vi "Measurement Logic.vi"() -> ()   [LabVIEW 2021, in "audio_intermodulationDistortionMeasurement.lvlib"]
uses:
  audio_intermodulationDistortionMeasurement.lvlib
  <vilib>/MeasurementLink/MeasurementLink Measurement Server/Classes/MeasurementContext/MeasurementContext.lvclass
  <vilib>/PDM Acquisition Toolkit/host/Classes/Tasks/PCM Input/Controls/DVR PCM Input Task.ctl
  <vilib>/PDM Acquisition Toolkit/host/Classes/Tasks/PCM Input/PCM Input Task.lvclass
  <vilib>/DAQmx/create/channels.llb/DAQmx Create Channel (AO-Voltage-Basic).vi
  <vilib>/DAQmx/configure/timing.llb/DAQmx Timing (Sample Clock).vi
  <vilib>/PDM Acquisition Toolkit/host/API/Public/Start/Start PCM Input Task.vi
  <vilib>/PDM Acquisition Toolkit/host/API/Public/Read/Read PCM Input Waveform.vi
  <vilib>/PDM Acquisition Toolkit/host/API/Public/Clear/Clear PCM Input Task.vi
  <resource>/objmgr/daqmx.rc
  <vilib>/PDM Acquisition Toolkit/host/API/PDM Acquisition Toolkit.lvlib
panel:
  out "Measurement Results":T1
  in  "Measurement Configuration":T2={"Analog Source Resource Name"="", "IMD Standard"=0, "Custom Low Frequency"=14000.0, "Custom High frequency"=15000.0, "Custom Amplitude Ratio"=1.0, "Amplitude"=-1.0, "Protocol Source Resource Name"="7821\\PCMi 0", "Input range"=2.825, "Number of Words"=19200, "Clock Rate"=12288000, "Latch Delay"=0.0} {"Custom Amplitude Ratio" format="%.1f"; "Custom High frequency" format="%_2p"; "Custom Low Frequency" format="%#_2p"; "Clock Rate" format="%.4p"}
  out "Measurement Context out":refnum<class "MeasurementContext.lvclass">
  in  "Measurement Context":refnum<class "MeasurementContext.lvclass">
  out "error out":errorcluster
  in  "error in":errorcluster
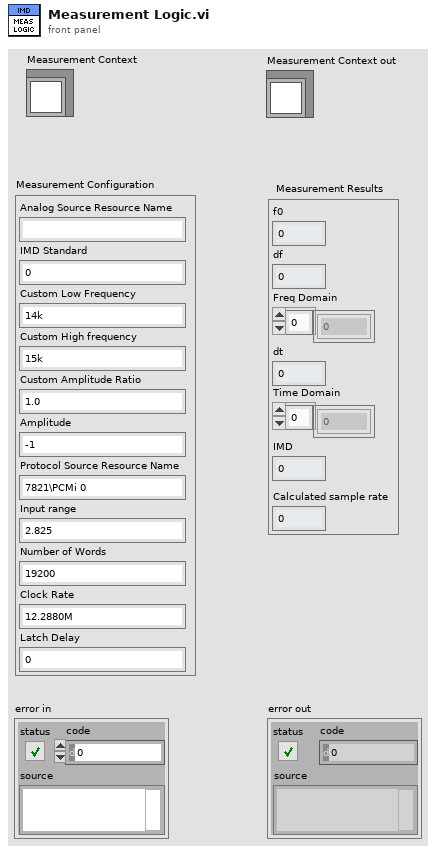
[diagram p1: front panel]
types:
  T1 = cluster{"f0":dbl, "df":dbl, "dt":dbl, "IMD":dbl, "Freq Domain":dbl[], "Time Domain":dbl[], "Calculated sample rate":u32}
  T2 = cluster{"Analog Source Resource Name":string, "IMD Standard":u16, "Custom Low Frequency":dbl, "Custom High frequency":dbl, "Custom Amplitude Ratio":dbl, "Amplitude":dbl, "Protocol Source Resource Name":string, "Input range":dbl, "Number of Words":i32, "Clock Rate":u32, "Latch Delay":dbl}
  T3 = typedef "PDM Acquisition Class Library.lvlib/PCM Input Task.lvclass/DVR PCM Input Task.ctl" = refnum<data-value>
  T4 = cluster{"task out":refnum<k21>, "SampClk.Rate":dbl, "PCM Input Task out":T3}
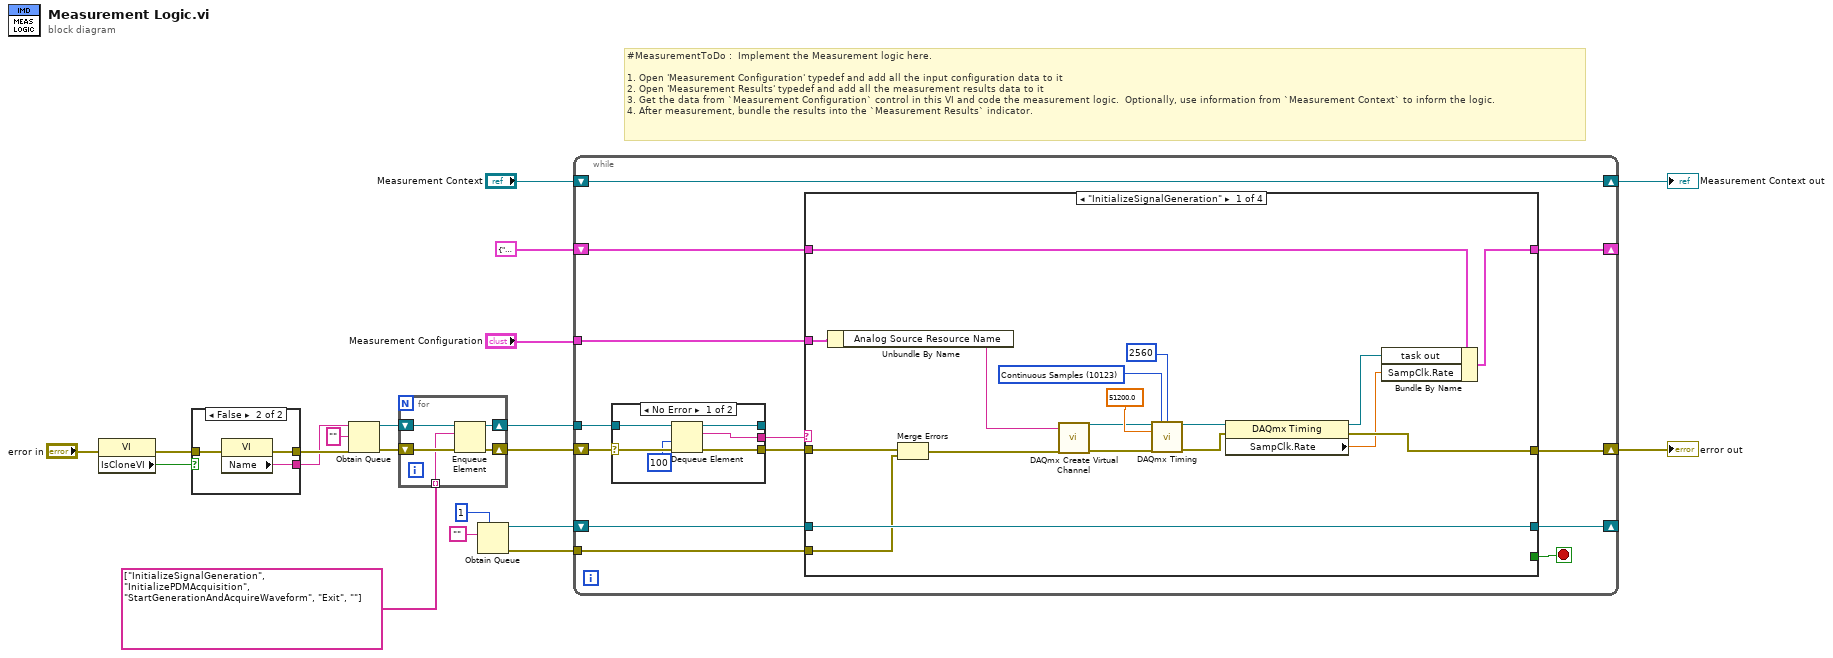
[diagram p0: block diagram]
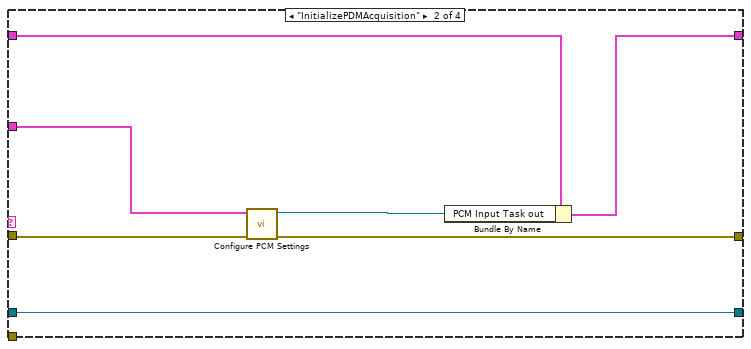
[diagram p2: hidden frame]
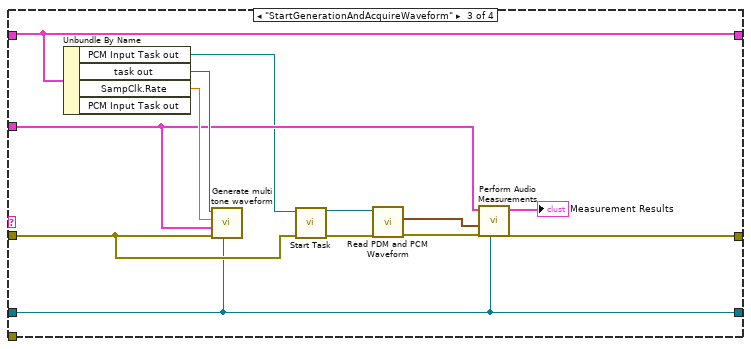
[diagram p3: hidden frame]
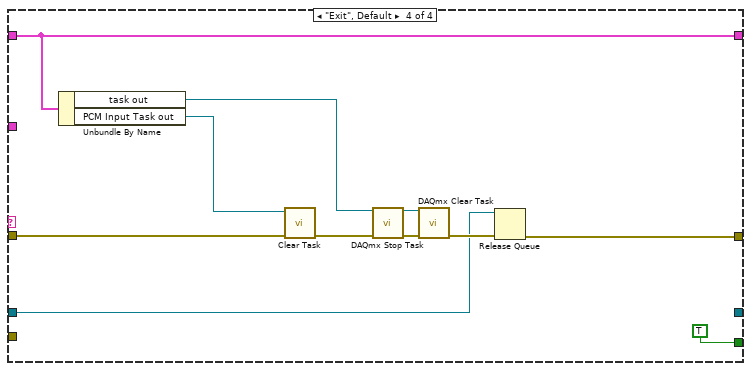
[diagram p4: hidden frame]
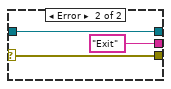
[diagram p5: hidden frame]
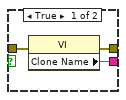
[diagram p6: hidden frame]
diagram:
  # "#MeasurementToDo :  Implement the Measurement logic here.\n\n1. Open 'Measurement Configuration' typedef and add all the input configuration data to it\n2. Open 'Measurement Results' typedef and add all the measurement results data to it\n3. Get the data from `Measurement Configuration` control in this VI and code the measurement logic.  Optionally, use information from `Measurement Context` to inform the logic.\n4. After measurement, bundle the results into the `Measurement Results` indicator."
  n1 = property class="VI"(error in="error in") -> (error out=w18:errorcluster, "IsCloneVI"=w19:bool)  [unwired: 1 in, 1 out]
  n2 = case shown="False" w19 {
    tunnel: [w23 w26] -> w17
    tunnel: [w22 w25] -> w16
    tunnel: w18 -> [w21 w24]
    frame True {
      n3 = property class="VI"(error in=w21) -> (error out=w23:errorcluster, "Clone Name"=w22:string)  [unwired: 1 in, 1 out]
    }
    frame False {
      n4 = property class="VI"(error in=w24) -> (error out=w26:errorcluster, "Name"=w25:string)  [unwired: 1 in, 1 out]
    }
  }
  n5 = Obtain Queue(name (unnamed)=w16, element data type="", error in (no error)=w17) -> (queue out=w13:refnum<queue>, error out=w14:errorcluster)  [unwired: 2 in, 1 out]
  n6 = for {
    shift-right: [w29] -> w7
    shift-left: w13 -> [w31]
    shift-right: [w28] -> w11
    shift-left: w14 -> [w30]
    tunnel: string[] ["InitializeSignalGeneration", "InitializePDMAcquisition", "StartGenerationAndAcquireWaveform", "Exit", ""] ("Step sequence") -> [w27] mode=indexing
    n7 = Enqueue Element(queue=w31, element=w27, error in (no error)=w30) -> (queue out=w29:refnum<queue>, error out=w28:errorcluster)  [unwired: 1 in, 1 out]
  }
  n8 = Obtain Queue(max queue size (-1, unlimited)=1, element data type="") -> (queue out=w2:refnum<queue>, error out=w3:errorcluster)  [unwired: 3 in, 1 out]
  n9 = while {
    shift-right: [w39] -> w10
    shift-left: w11 -> [w44]
    shift-right: [w41] -> w8
    shift-left: "Measurement Context" -> [w41]
    tunnel: w7 -> [w43]
    tunnel: "Measurement Configuration" -> [w37]
    shift-right: [w36] -> _
    shift-left: T4 {"task out"="", "SampClk.Rate"=0.0, "PCM Input Task out"=refnum} -> [w32]
    tunnel: w3 -> [w35]
    shift-right: [w33] -> _
    shift-left: w2 -> [w34]
    stop <- w38 stop-if-true
    n10 = case shown="No Error" w44 {
      selector: w44 -> [w97 w101]
      tunnel: w43 -> [w99 w100]
      tunnel: [w98 "Exit" ("t")] -> w42
      tunnel: [w96 w101] -> w40
      tunnel: [w94 w100] -> _
      frame No Error {
        n11 = Dequeue Element(queue=w99, timeout in ms (-1)=100, error in (no error)=w97) -> (queue out=w94:refnum<queue>, element=w98:string, error out=w96:errorcluster)  [unwired: 1 out]
      }
      frame Error {
      }
    }
    n12 = case shown="\"InitializeSignalGeneration\"" w42 {
      tunnel: w40 -> [w45 w65 w74 w92]
      tunnel: [w58 w64 w80 w84] -> w39
      tunnel: [_ _ _ TRUE] -> w38
      tunnel: w37 -> [w59 w66 w75 _]
      tunnel: w32 -> [w52 w69 w71 w88]
      tunnel: [w49 w68 w71 w88] -> w36
      tunnel: w35 -> [w46 _ _ _]
      tunnel: w34 -> [w48 w67 w73 w83]
      tunnel: [w48 w67 w73 _] -> w33
      frame "InitializeSignalGeneration" {
        w56 = 10123 items=["Finite Samples"=10178, "Continuous Samples"=10123, "Hardware Timed Single Point"=12522] ("sample mode")
        n13 = Unbundle By Name(w59) -> ("Analog Source Resource Name"=w60:string)
        n14 = Merge Errors(w45, w46) -> (w47:errorcluster)
        n15 = call-poly <vilib>:"DAQmx Create Virtual Channel.vi"("physical channels"=w60, "error in"=w47) -> ("task out"=w53:refnum<k21>, "error out"=w62:errorcluster)  [unwired: 12 in]
        n16 = call-poly <vilib>:"DAQmx Timing.vi"("task/channels in"=w53, "sample mode"=w56, "samples per channel"=2560, "rate"=51200.0, "error in"=w62) -> ("task out"=w54:refnum<k21>, "error out"=w61:errorcluster)  [unwired: 9 in]
        n17 = property class="DAQmx Timing"(reference=w54, error in=w61) -> (reference out=w50:refnum<k21>, error out=w58:errorcluster, "SampClk.Rate"=w51:dbl)
        n18 = Bundle By Name(cluster=w52, "task out"=w50, "SampClk.Rate"=w51) -> (w49:T4)
      }
      frame "InitializePDMAcquisition" {
        n19 = call "Configure PCM Settings.vi"("error in"=w65, "Measurement Configuration"=w66) -> ("error out"=w64:errorcluster, "PCM Input Task out"=w63:T3)  [unwired: 8 in]
        n20 = Bundle By Name(cluster=w69, "PCM Input Task out"=w63) -> (w68:T4)
      }
      frame "StartGenerationAndAcquireWaveform" {
        n21 = Unbundle By Name(w71) -> ("PCM Input Task out"=w72:T3, "task out"=w76:refnum<k21>, "SampClk.Rate"=w77:dbl)  [unwired: 1 out]
        n22 = call "Generate multi tone waveform.vi"("queue"=w73, "error in"=w74, "Measurement Configuration"=w75, "Sample Rate (Hz)"=w77, "task/channels in"=w76) -> ()  [unwired: 5 in, 2 out]
        n23 = call-poly <vilib>:"Start Task.vi"("error in"=w74, "PCM input task in"=w72) -> ("error out"=w82:errorcluster, "PCM input task out"=w78:T3)  [unwired: 8 in]
        n24 = call-poly <vilib>:"Read PDM and PCM Waveform.vi"("error in"=w82, "PCM input task In"=w78) -> ("error out"=w81:errorcluster, "PCM waveforms"=w79:waveform(dbl)[])  [unwired: 4 in, 4 out]
        n25 = call "Perform Audio Measurements.vi"("queue"=w73, "error in"=w81, "PCM waveforms"=w79, "Measurement Configuration"=w75) -> ("error out"=w80:errorcluster, "Measurement Results"=→"Measurement Results":T1)  [unwired: 6 in]
      }
      frame "Exit", Default {
        n26 = Unbundle By Name(w88) -> ("task out"=w86:refnum<k21>, "PCM Input Task out"=w87:T3)
        n27 = call-poly <vilib>:"Clear Task.vi"("error in"=w92, "PCM input task in"=w87) -> ("error out"=w91:errorcluster)  [unwired: 9 in]
        n28 = call <vilib>:"DAQmx Stop Task.vi"("task/channels in"=w86, "error in"=w91) -> ("task out"=w89:refnum<k21>, "error out"=w90:errorcluster)  [unwired: 12 in]
        n29 = call <vilib>:"DAQmx Clear Task.vi"("task in"=w89, "error in"=w90) -> ("error out"=w85:errorcluster)  [unwired: 13 in]
        n30 = Release Queue(queue=w83, error in (no error)=w85) -> (error out=w84:errorcluster)  [unwired: 1 in, 2 out]
      }
    }
  }
  "error out" <- w10
  "Measurement Context out" <- w8
